vi "_055.vi"() -> ()   [LabVIEW 2024]
panel:
  out "sum":i16
  in  "String 2":string
  out "length":i32
  out "String":string
  out "error out":errorcluster
  in  "Path":path
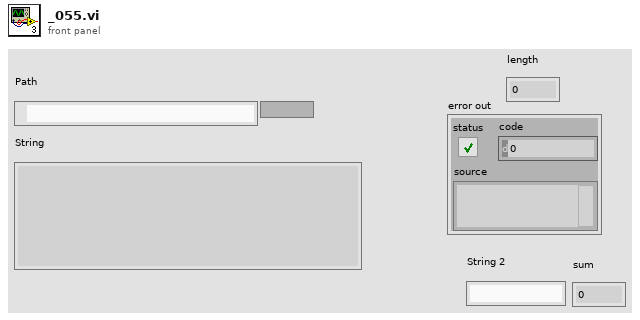
[diagram p1: front panel]
types:
  T1 = enum16{"open", "replace", "create", "open or create", "replace or create", "replace or create with confirmation"}
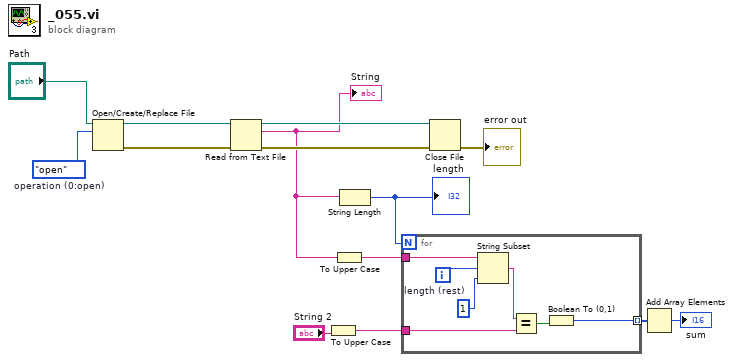
[diagram p0: block diagram]
diagram:
  w8 = T1."open"  # operation (0:open)
  n1 = Open/Create/Replace File(file path (use dialog)="Path", operation (0:open)=w8) -> (refnum out=w14:refnum<file>, error out=w12:errorcluster)  [unwired: 4 in, 1 out]
  n2 = Read from Text File(file (use dialog)=w14, error in=w12) -> (refnum out=w13:refnum<file>, text=w7:string, error out=w11:errorcluster)  [unwired: 2 in, 1 out]
  "String" <- w7
  n3 = To Upper Case(1:"String 2") -> (0:w3:string)
  n4 = To Upper Case(1:w7) -> (0:w5:string)
  n5 = String Length(string=w7) -> (length=w6:i32)
  "length" <- w6
  n6 = for {
    N: w6 -> [_]
    tunnel: w5 -> [w21]
    tunnel: w3 -> [w18]
    tunnel: [w15] -> w2 mode=indexing
    i -> [w20]
    w19 = 1  # length (rest)
    n7 = String Subset(string=w21, offset (0)=w20, length (rest)=w19) -> (substring=w17:string)
    n8 = Equal?(x=w17, y=w18) -> (x = y?=w16:bool)
    n9 = Boolean To (0,1)(Boolean=w16) -> (0, 1=w15:i16)
  }
  n10 = Close File(refnum=w13, error in=w11) -> (error out=→"error out":errorcluster)  [unwired: 1 out]
  n11 = Add Array Elements(numeric array=w2) -> (sum=→"sum":i16)
